vi "scroll.vi"(1 "Array":string[][](array[string]), 2 "Numeric in":i32) -> (0 "Numeric out":i32)   [LabVIEW 2015]
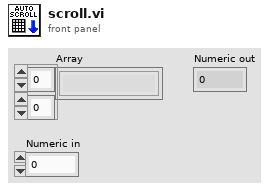
[diagram p1: front panel]
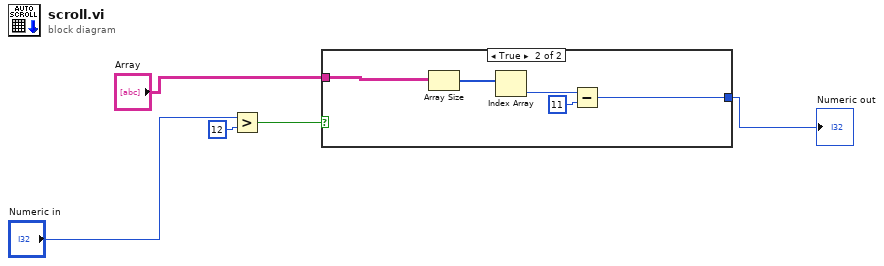
[diagram p0: block diagram]
diagram:
  n1 = Greater?(x="Numeric in", y=12) -> (0:w4:bool)
  n2 = case shown="True" w4 {
    tunnel: "Array" -> [_ w7]
    tunnel: [_ w6] -> w5
    frame False {
    }
    frame True {
      n3 = Array Size(array=w7) -> (size(s)=w10:i32[])
      n4 = Index Array(array=w10) -> (element=w9:i32)  [unwired: 1 in]
      n5 = Subtract(x=w9, y=11) -> (x-y=w6:i32)
    }
  }
  "Numeric out" <- w5
